vi "Close Progress Bar.vi"(8 "error in (no error)":errorcluster, 11 "Progress Bar Dialog":refnum<class "Loading Dialog.lvclass">) -> (0 "error out":errorcluster)   [LabVIEW 2020, in "VI Properties Editor.lvlib" / "Loading Dialog.lvclass"]
doc: "This VI increments the progress bar one final time and closes the references associated with the progress bar."
uses:
  Loading Dialog.lvclass
  Loading Dialog.lvclass/Loading Dialog.ctl
panel:
  in  "Load Complete":string="Load Complete"
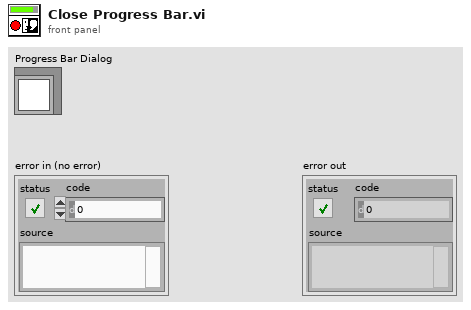
[diagram p1: front panel]
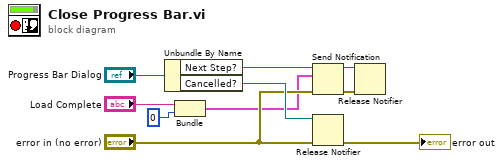
[diagram p0: block diagram]
diagram:
  n1 = Unbundle By Name("Progress Bar Dialog") -> ("Next Step?"=w7:refnum<notifier>, "Cancelled?"=w6:refnum<notifier>)
  n2 = Bundle("Load Complete"="Load Complete", 0) -> (w1:cluster{"Load Complete":string, i32})  [unwired: 1 in]
  n3 = Send Notification(notification=w1, notifier=w7, error in (no error)="error in (no error)") -> (notifier out=w9:refnum<notifier>, error out=w10:errorcluster)
  n4 = Release Notifier(notifier=w6, error in (no error)="error in (no error)") -> (error out=→"error out":errorcluster)  [unwired: 1 in, 2 out]
  n5 = Release Notifier(notifier=w9, error in (no error)=w10) -> ()  [unwired: 1 in, 3 out]
